vi "myCommOut.vi"(0 "Modbus Master输入":refnum<class "Modbus Master.lvclass">, 1 "freqs行":i32[](array[numeric]), 3 "默认幅值 Amp0":u8(ring)=2 items=["10.0", "5.0", "1.0", "0.5", "0.1", "0.05", "0.01"], 5 "地址":u16, 6 "实际幅值 Amp":u8(ring)=1 items=["= Amp0", "= Amp0 / freq"], 7 "t_wait":dbl=0.04, 9 "扰动注入模式":i32(ring) items=["无注入", "单相注入", "d轴注入", "q轴注入", "正(负)序注入"], 10 "最大同时扫频数":u32=5 min=1 max=10, 11 "错误输入（无错误）":errorcluster, 12 "基波频率":u32=50, 13 "单相注入至":u8(ring) items=["A相或直流", "B相", "C相"]) -> (4 "Modbus Master输出":refnum<class "Modbus Master.lvclass">, 8 "error out":bool, 15 "错误输出":errorcluster)   [LabVIEW 2024]
uses:
  <vilib>/NI/Modbus Library/API/Master/Modbus Master.lvclass
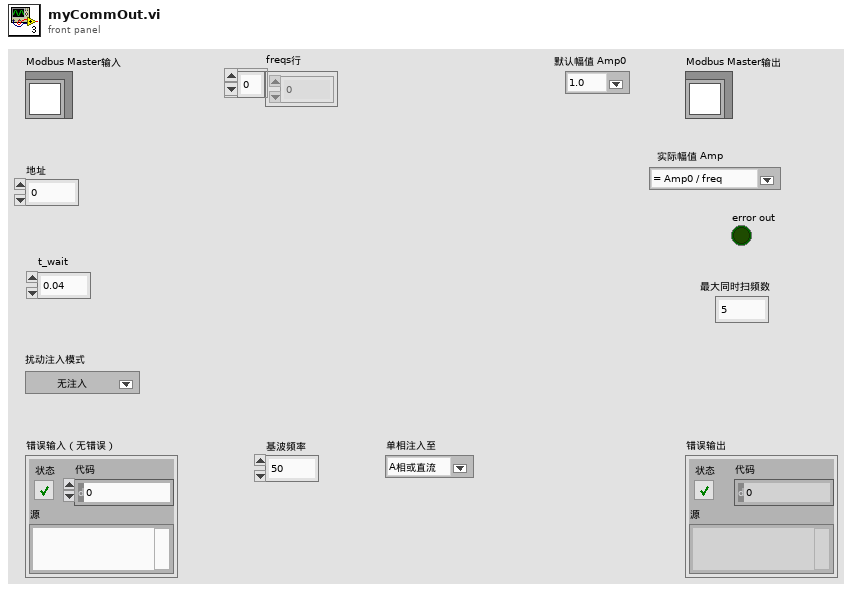
[diagram p1: front panel]
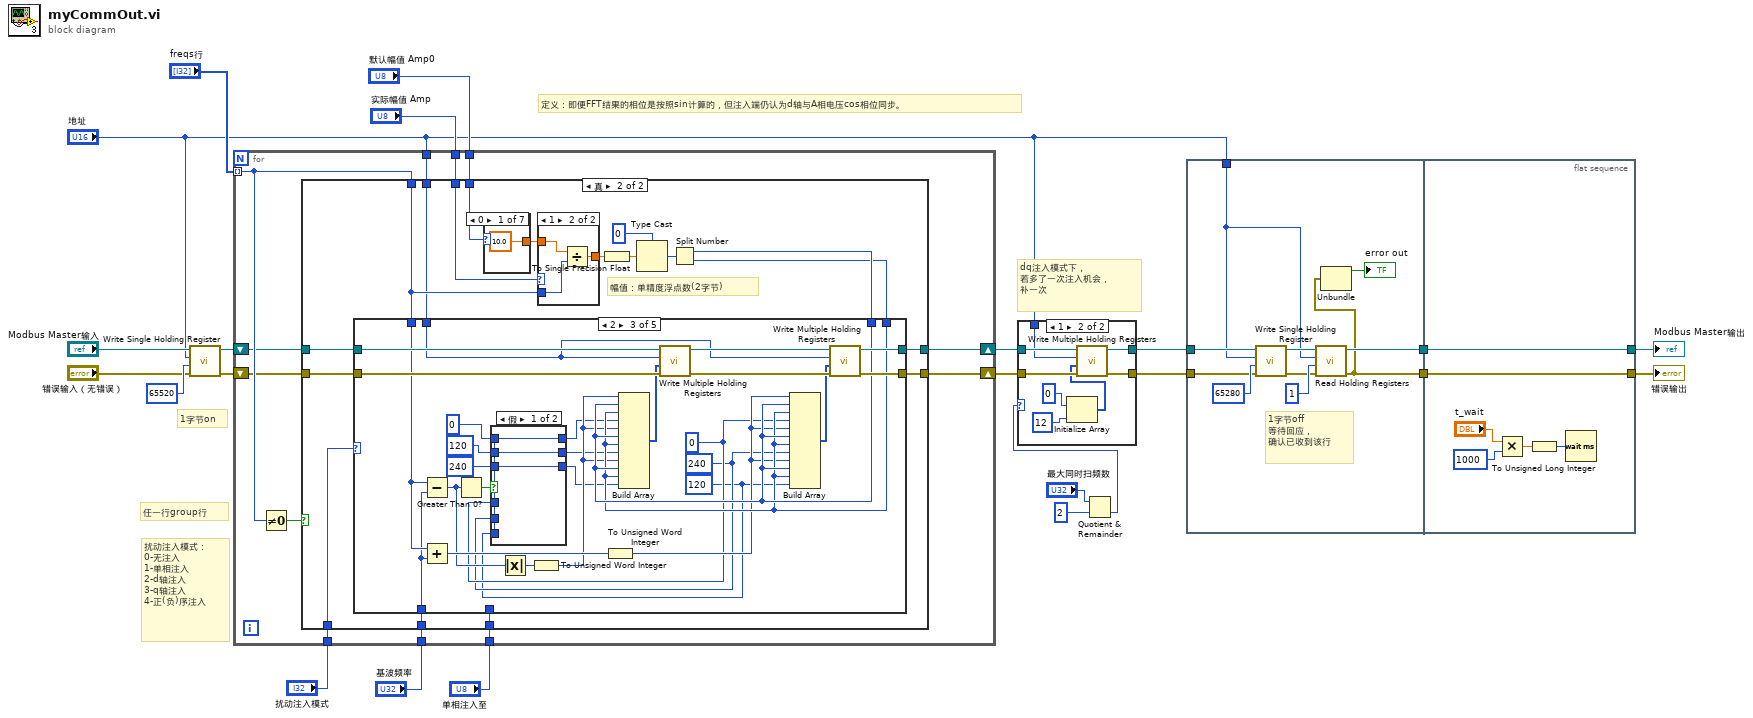
[diagram p0: block diagram]
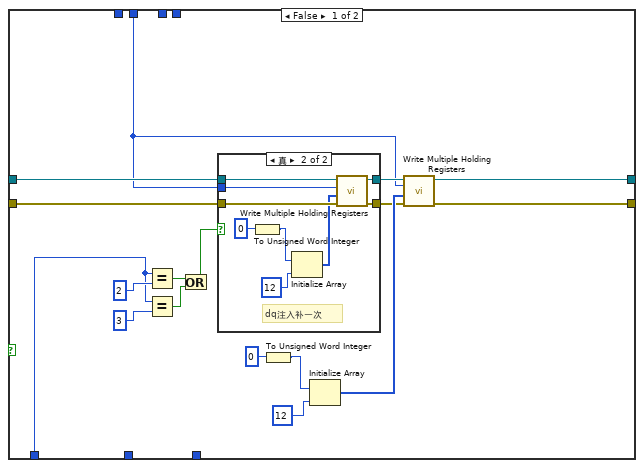
[diagram p3: hidden frame]
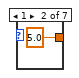
[diagram p6: hidden frame]
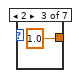
[diagram p7: hidden frame]
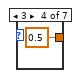
[diagram p8: hidden frame]
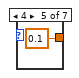
[diagram p9: hidden frame]
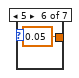
[diagram p10: hidden frame]
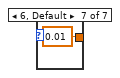
[diagram p11: hidden frame]
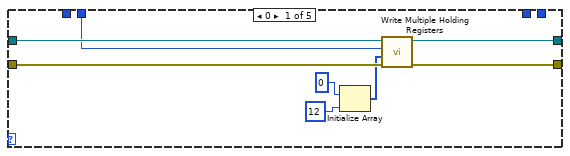
[diagram p12: hidden frame]
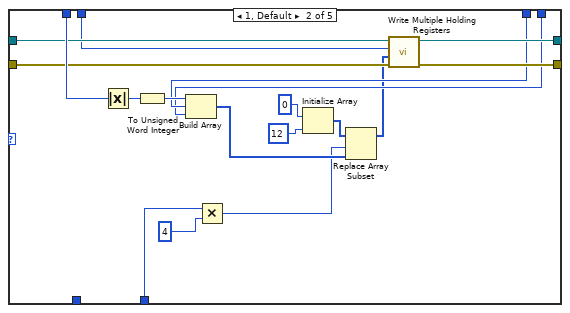
[diagram p13: hidden frame]
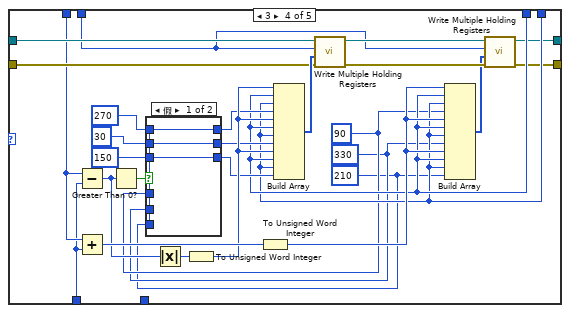
[diagram p15: hidden frame]
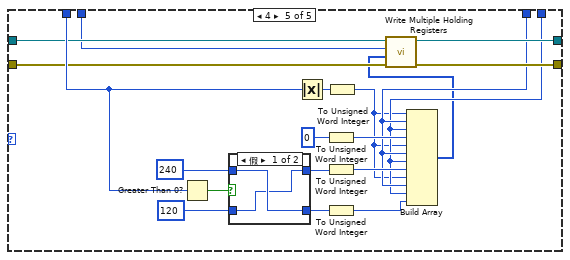
[diagram p17: hidden frame]
diagram:
  # "定义：即便FFT结果的相位是按照sin计算的，但注入端仍认为d轴与A相电压cos相位同步。"
  # "dq注入模式下，\n若多了一次注入机会，\n补一次"
  # "扰动注入模式：\n0-无注入\n1-单相注入\n2-d轴注入\n3-q轴注入\n4-正(负)序注入"
  # "任一行group行"
  # "1字节on"
  n1 = call-dynamic "Write Single Holding Register.vi"("error in"="错误输入（无错误）", "register to write"=u16 65520, "address"="地址", "Modbus master in"="Modbus Master输入") -> ("error out"=w12:errorcluster, "Modbus master out"=w11:refnum<class "Modbus Master.lvclass">)  [unwired: 6 in]
  n2 = for {
    shift-right: [w31] -> w16
    shift-left: w11 -> [w33]
    shift-right: [w30] -> w17
    shift-left: w12 -> [w32]
    tunnel: "freqs行" -> [w35] mode=indexing
    tunnel: "地址" -> [w29]
    tunnel: "扰动注入模式" -> [w28]
    tunnel: "实际幅值 Amp" -> [w27]
    tunnel: "默认幅值 Amp0" -> [w26]
    tunnel: "基波频率" -> [w25]
    tunnel: "单相注入至" -> [w24]
    n3 = Not Equal To 0?(x=w35) -> (x != 0?=w34:bool)
    n4 = case shown="真" w34 {
      tunnel: w35 -> [_ w81]
      tunnel: [w49 w69] -> w30
      tunnel: w33 -> [w45 w73]
      tunnel: [w48 w70] -> w31
      tunnel: w32 -> [w46 w72]
      tunnel: w29 -> [w42 w71]
      tunnel: w28 -> [w36 w68]
      tunnel: w27 -> [_ w67]
      tunnel: w26 -> [_ w66]
      tunnel: w25 -> [_ w65]
      tunnel: w24 -> [_ w64]
      frame False {
        n5 = Equal?(x=w36, y=2) -> (x = y?=w38:bool)
        n6 = Equal?(x=w36, y=3) -> (x = y?=w39:bool)
        n7 = Or(x=w38, y=w39) -> (x .or. y?=w37:bool)
        n8 = case shown="真" w37 {
          tunnel: w46 -> [w53 w63]
          tunnel: w45 -> [w54 w62]
          tunnel: [w54 w61] -> w44
          tunnel: [w53 w60] -> w43
          tunnel: w42 -> [_ w55]
          frame False {
          }
          frame True {
            # "dq注入补一次"
            n9 = To Unsigned Word Integer(number=u16 0) -> (unsigned 16bit integer=w58:u16)
            n10 = Initialize Array(w58, 12 ("维数大小")) -> (w56:u16[])
            n11 = call-dynamic "Write Multiple Holding Registers.vi"("error in"=w63, "registers to write"=w56, "starting address"=w55, "Modbus master in"=w62) -> ("error out"=w60:errorcluster, "Modbus master out"=w61:refnum<class "Modbus Master.lvclass">)  [unwired: 6 in]
          }
        }
        n12 = To Unsigned Word Integer(number=u16 0) -> (unsigned 16bit integer=w51:u16)
        n13 = Initialize Array(w51, 12 ("维数大小")) -> (w47:u16[])
        n14 = call-dynamic "Write Multiple Holding Registers.vi"("error in"=w43, "registers to write"=w47, "starting address"=w42, "Modbus master in"=w44) -> ("error out"=w49:errorcluster, "Modbus master out"=w48:refnum<class "Modbus Master.lvclass">)  [unwired: 6 in]
      }
      frame True {
        # "幅值：单精度浮点数(2字节)"
        n15 = case shown="0" w66 {
          tunnel: [10.0 5.0 1.0 0.5 0.1 0.05 0.01] -> w80
          frame 0 {
          }
          frame 1 {
          }
          frame 2 {
          }
          frame 3 {
          }
          frame 4 {
          }
          frame 5 {
          }
          frame 6, Default {
          }
        }
        n16 = case shown="1" w67 {
          tunnel: w80 -> [w82 w85]
          tunnel: w81 -> [_ w84]
          tunnel: [w82 w83] -> w78
          frame 0, Default {
          }
          frame 1 {
            n17 = Divide(x=w85, y=w84) -> (x/y=w83:dbl)
          }
        }
        n18 = To Single Precision Float(number=w78) -> (single precision float=w79:sgl)
        n19 = Type Cast(type=0, x=w79) -> (*(type *) &x=w76:i32)
        n20 = Split Number(x=w76) -> (hi(x)=w75:u16, lo(x)=w74:u16)
        n21 = case shown="2" w68 {
          tunnel: w81 -> [_ w117 w137 w165 w199]
          tunnel: w75 -> [_ w108 w139 w163 w190]
          tunnel: w74 -> [_ w107 w138 w162 w189]
          tunnel: [w98 w112 w141 w161 w196] -> w70
          tunnel: w73 -> [w96 w115 w145 w167 w198]
          tunnel: [w97 w113 w140 w160 w195] -> w69
          tunnel: w72 -> [w95 w116 w144 w166 w197]
          tunnel: w71 -> [w94 w114 w123 w164 w194]
          tunnel: w65 -> [_ _ w119 w153 _]
          tunnel: w64 -> [_ w101 _ _ _]
          frame 0 {
            n22 = Initialize Array(u16 0, 12 ("维数大小")) -> (w93:u16[])
            n23 = call-dynamic "Write Multiple Holding Registers.vi"("error in"=w95, "registers to write"=w93, "starting address"=w94, "Modbus master in"=w96) -> ("error out"=w97:errorcluster, "Modbus master out"=w98:refnum<class "Modbus Master.lvclass">)  [unwired: 6 in]
          }
          frame 1, Default {
            n24 = Absolute Value(x=w117) -> (abs(x)=w118:i32)
            n25 = To Unsigned Word Integer(number=w118) -> (unsigned 16bit integer=w109:u16)
            n26 = Build Array(w109, w108, w107) -> (w105:u16[])
            n27 = Multiply(x=w101, y=4 ("索引")) -> (x*y=w102:i32)
            n28 = Initialize Array(u16 0, 12 ("维数大小")) -> (w106:u16[])
            n29 = Replace Array Subset(array=w106, new element=w105, index=w102) -> (w104:u16[])
            n30 = call-dynamic "Write Multiple Holding Registers.vi"("error in"=w116, "registers to write"=w104, "starting address"=w114, "Modbus master in"=w115) -> ("error out"=w113:errorcluster, "Modbus master out"=w112:refnum<class "Modbus Master.lvclass">)  [unwired: 6 in]
          }
          frame 2 {
            w120 = u16 120
            w121 = u16 240
            w122 = u16 0
            n31 = Subtract(x=w137, y=w119) -> (x-y=w134:u32)
            n32 = Add(x=w137, y=w119) -> (x+y=w136:u32)
            n33 = Greater Than 0?(x=w134) -> (x > 0?=w132:bool)
            n34 = case shown="假" w132 {
              tunnel: u16 0 -> [_ w152]
              tunnel: u16 120 -> [_ w151]
              tunnel: u16 240 -> [_ w150]
              tunnel: [w149 w152] -> w128
              tunnel: [w148 w151] -> w127
              tunnel: [w147 w150] -> w126
              tunnel: w122 -> [w149 _]
              tunnel: w121 -> [w148 _]
              tunnel: w120 -> [w147 _]
              frame False {
              }
              frame True {
              }
            }
            n35 = Absolute Value(x=w134) -> (abs(x)=w146:i32)
            n36 = To Unsigned Word Integer(number=w146) -> (unsigned 16bit integer=w133:u16)
            n37 = To Unsigned Word Integer(number=w136) -> (unsigned 16bit integer=w135:u16)
            n38 = Build Array(w133, w139, w138, w128, w133, w139, w138, w127, w133, w139, w138, w126) -> (w125:u16[])
            n39 = call-dynamic "Write Multiple Holding Registers.vi"("error in"=w144, "registers to write"=w125, "starting address"=w123, "Modbus master in"=w145) -> ("error out"=w142:errorcluster, "Modbus master out"=w143:refnum<class "Modbus Master.lvclass">)  [unwired: 6 in]
            n40 = Build Array(w135, w139, w138, w122, w135, w139, w138, w121, w135, w139, w138, w120) -> (w124:u16[])
            n41 = call-dynamic "Write Multiple Holding Registers.vi"("error in"=w142, "registers to write"=w124, "starting address"=w123, "Modbus master in"=w143) -> ("error out"=w140:errorcluster, "Modbus master out"=w141:refnum<class "Modbus Master.lvclass">)  [unwired: 6 in]
          }
          frame 3 {
            w157 = u16 210
            w158 = u16 330
            w159 = u16 90
            n42 = Subtract(x=w165, y=w153) -> (x-y=w175:u32)
            n43 = Add(x=w165, y=w153) -> (x+y=w177:u32)
            n44 = Greater Than 0?(x=w175) -> (x > 0?=w173:bool)
            n45 = case shown="假" w173 {
              tunnel: u16 270 -> [_ w186]
              tunnel: u16 30 -> [_ w185]
              tunnel: u16 150 -> [_ w184]
              tunnel: [w183 w186] -> w172
              tunnel: [w182 w185] -> w171
              tunnel: [w181 w184] -> w170
              tunnel: w159 -> [w183 _]
              tunnel: w158 -> [w182 _]
              tunnel: w157 -> [w181 _]
              frame False {
              }
              frame True {
              }
            }
            n46 = Absolute Value(x=w175) -> (abs(x)=w180:i32)
            n47 = To Unsigned Word Integer(number=w180) -> (unsigned 16bit integer=w174:u16)
            n48 = To Unsigned Word Integer(number=w177) -> (unsigned 16bit integer=w176:u16)
            n49 = Build Array(w174, w163, w162, w172, w174, w163, w162, w171, w174, w163, w162, w170) -> (w169:u16[])
            n50 = call-dynamic "Write Multiple Holding Registers.vi"("error in"=w166, "registers to write"=w169, "starting address"=w164, "Modbus master in"=w167) -> ("error out"=w178:errorcluster, "Modbus master out"=w179:refnum<class "Modbus Master.lvclass">)  [unwired: 6 in]
            n51 = Build Array(w176, w163, w162, w159, w176, w163, w162, w158, w176, w163, w162, w157) -> (w168:u16[])
            n52 = call-dynamic "Write Multiple Holding Registers.vi"("error in"=w178, "registers to write"=w168, "starting address"=w164, "Modbus master in"=w179) -> ("error out"=w160:errorcluster, "Modbus master out"=w161:refnum<class "Modbus Master.lvclass">)  [unwired: 6 in]
          }
          frame 4 {
            n53 = Greater Than 0?(x=w199) -> (x > 0?=w204:bool)
            n54 = case shown="假" w204 {
              tunnel: [w207 w210] -> w203
              tunnel: u16 240 -> [w208 w210]
              tunnel: [w208 w209] -> w201
              tunnel: 120 -> [w207 w209]
              frame False {
              }
              frame True {
              }
            }
            n55 = Absolute Value(x=w199) -> (abs(x)=w206:i32)
            n56 = To Unsigned Word Integer(number=u16 0) -> (unsigned 16bit integer=w193:u16)
            n57 = To Unsigned Word Integer(number=w203) -> (unsigned 16bit integer=w191:u16)
            n58 = To Unsigned Word Integer(number=w201) -> (unsigned 16bit integer=w192:u16)
            n59 = To Unsigned Word Integer(number=w206) -> (unsigned 16bit integer=w188:u16)
            n60 = Build Array(w188, w190, w189, w193, w188, w190, w189, w191, w188, w190, w189, w192) -> (w187:u16[])
            n61 = call-dynamic "Write Multiple Holding Registers.vi"("error in"=w197, "registers to write"=w187, "starting address"=w194, "Modbus master in"=w198) -> ("error out"=w195:errorcluster, "Modbus master out"=w196:refnum<class "Modbus Master.lvclass">)  [unwired: 6 in]
          }
        }
      }
    }
  }
  n62 = Quotient & Remainder(x="最大同时扫频数", y=u32 2) -> (floor(x/y)=w18:u32)  [unwired: 1 out]
  n63 = case shown="1" w18 {
    tunnel: [w212 w217] -> w7
    tunnel: w16 -> [w212 w220]
    tunnel: [w211 w218] -> w6
    tunnel: w17 -> [w211 w219]
    tunnel: "地址" -> [_ w213]
    frame 0, Default {
    }
    frame 1 {
      n64 = Initialize Array(u16 0, 12 ("维数大小")) -> (w214:u16[])
      n65 = call-dynamic "Write Multiple Holding Registers.vi"("error in"=w219, "registers to write"=w214, "starting address"=w213, "Modbus master in"=w220) -> ("error out"=w218:errorcluster, "Modbus master out"=w217:refnum<class "Modbus Master.lvclass">)  [unwired: 6 in]
    }
  }
  n66 = flat-sequence {
    tunnel: w7 -> [w225]
    tunnel: w6 -> [w224]
    tunnel: "地址" -> [w221]
    tunnel: [w223] -> w2
    tunnel: [w222] -> w1
    tunnel: [w235] -> w4
    tunnel: [w236] -> w5
    tunnel: w2 -> [w236]
    tunnel: w1 -> [w235]
    frame #0 {
      # "1字节off\n等待回应，\n确认已收到该行"
      n67 = call-dynamic "Write Single Holding Register.vi"("error in"=w224, "register to write"=u16 65280, "address"=w221, "Modbus master in"=w225) -> ("error out"=w227:errorcluster, "Modbus master out"=w228:refnum<class "Modbus Master.lvclass">)  [unwired: 6 in]
      n68 = call-dynamic "Read Holding Registers.vi"("error in"=w227, "number of inputs"=u16 1, "starting address"=w221, "Modbus master in"=w228) -> ("error out"=w222:errorcluster, "Modbus master out"=w223:refnum<class "Modbus Master.lvclass">)  [unwired: 5 in, 1 out]
      n69 = Unbundle(w222) -> ("status"=→"error out":bool)  [unwired: 2 out]
    }
    frame #1 {
      n70 = Multiply(x="t_wait", y=1000) -> (x*y=w233:dbl)
      n71 = To Unsigned Long Integer(number=w233) -> (unsigned 32bit integer=w232:u32)
      n72 = Wait (ms)(milliseconds to wait=w232) -> ()  [unwired: 1 out]
    }
  }
  "错误输出" <- w4
  "Modbus Master输出" <- w5
